vi "Teleop.vi"(10 "Match Info":T2={"Autonomous Elapsed Seconds"=0.0, "TeleOp Elapsed Seconds"=59.421, "Disabled Elapsed Seconds"=50.178, "Visited Autonomous"=FALSE, "Visited TeleOp"=TRUE, "Visited Disabled"=TRUE, "Autonomous Settings"={"Autonomous Style"=enum."Independent", "VI Refnum"=refnum}}, 11 "Call Context":T3=enum."Stop") -> ()   [LabVIEW 2014]
doc: "This VI is called for each TeleOp packet received from the DS where the robot is not disabled. It is often used to read from the joysticks and update I/O or to update setpoints for timed control loops. It should complete and return within 20 milliseconds or it may miss DS packets."
uses:
  <vilib>/Rock Robotics/WPI/DriverStation/WPI_DriverStationDerivedRobotMode.ctl
  <vilib>/Rock Robotics/WPI/DriverStation/WPI_DriverStationMatch Info.ctl
  <vilib>/Rock Robotics/WPI/RobotDrive/WPI_RobotDriveGetSetRefNum.vi
  <vilib>/Rock Robotics/WPI/Joystick/WPI_JoystickGetSetRefNum.vi
  <vilib>/Rock Robotics/Network Tables/SD Write Numeric Array.vi
  <vilib>/Rock Robotics/Network Tables/SD Write Boolean Array.vi
  Robot Global Data.vi
  <vilib>/Rock Robotics/WPI/RobotDrive/WPI_RobotDriveMecanumDrive_Cartesian.vi
panel:
  out "North":dbl
  out "current (A)":dbl(graph)
  in  "Clear Sticky Faults":bool
  in  "PID gains":T1={"proportional gain (Kc)"=0.021, "integral time (Ti, min)"=0.0, "derivative time (Td, min)"=0.0} {"derivative time (Td, min)" format="%.3f"; "integral time (Ti, min)" format="%.3f"; "proportional gain (Kc)" format="%.3f"}
  # "EDITED: 3/8/15"
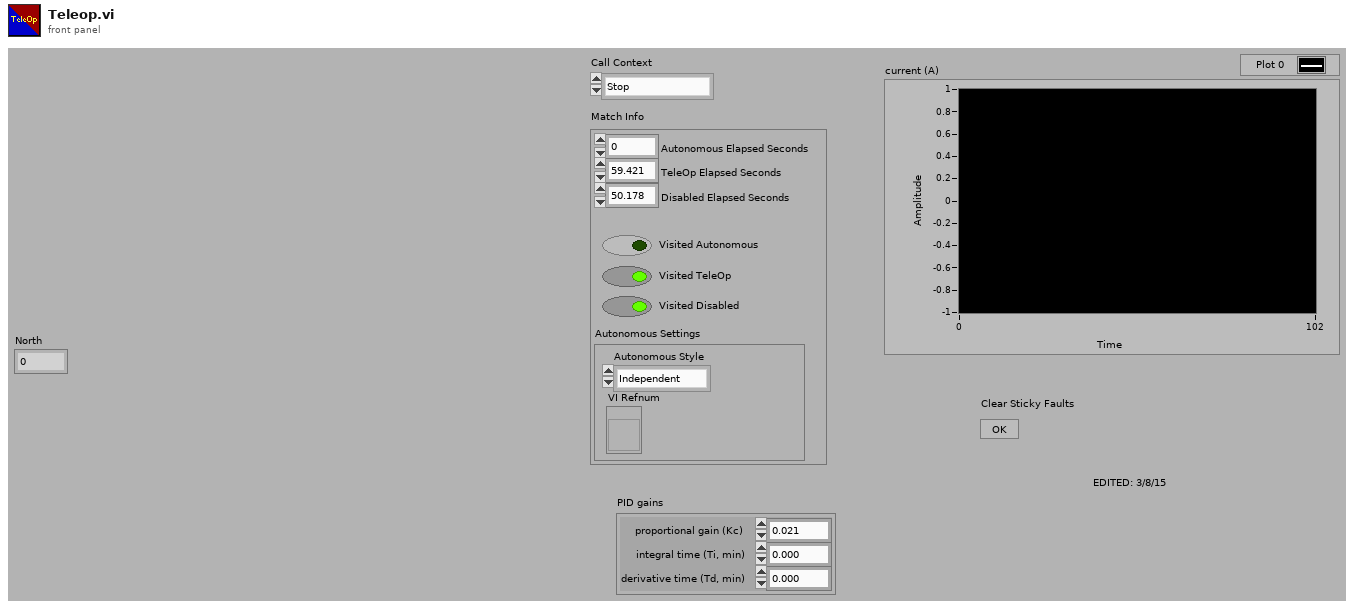
[diagram p1: front panel]
types:
  T1 = cluster{"proportional gain (Kc)":dbl, "integral time (Ti, min)":dbl, "derivative time (Td, min)":dbl}
  T2 = typedef "WPI_DriverStationMatch Info.ctl" = cluster{"Autonomous Elapsed Seconds":dbl, "TeleOp Elapsed Seconds":dbl, "Disabled Elapsed Seconds":dbl, "Visited Autonomous":bool, "Visited TeleOp":bool, "Visited Disabled":bool, "Autonomous Settings":cluster{"Autonomous Style":enum16{"Iterative", "Independent"}, "VI Refnum":refnum<vi>}}
  T3 = typedef "WPI_DriverStationDerivedRobotMode.ctl" = enum16{"Init", "Execute", "Stop"}
  T4 = typedef "WPI_JoystickDevRef.ctl" = cluster{"Device":T5}
  T5 = typedef "WPI_JoystickDeviceEnum.ctl" = enum16{"USB 0", "USB 1", "USB 2", "USB 3", "USB 4", "USB 5"}
  T6 = typedef "WPI_RobotDriveDevRef.ctl" = cluster{"DevStatus":errorcluster, "Motors[]":T7[], "Square Inputs":bool, "Max Output":dbl}
  T7 = typedef "WPI_MotorControlDeviceRef.ctl" = cluster{"DeviceStatus":errorcluster, "Type":T8, "PWM":cluster{"Controller":T9, "PWM Channel":T10, "DeadBand":T11}, "CAN":cluster{"Device Number":u8, "Control Mode":T12, "Semaphore":T13, "Max Vout":dbl, "TalonSRX Control Mode":T14}, "Invert":bool, "TransformRef":T15, "InvTransformRef":T15}
  T8 = typedef "WPI_MotorControlType.ctl" = enum16{"PWM", "CAN", "CANTalonSRX"}
  T9 = typedef "FPGA_TypedefDigitalModule.ctl" = enum16{"Controller 1"}
  T10 = typedef "FPGA_DIOPWMChannel.ctl" = enum8{"PWM 0", "PWM 1", "PWM 2", "PWM 3", "PWM 4", "PWM 5", "PWM 6", "PWM 7", "PWM 8", "PWM 9", "PWM MXP 0", "PWM MXP 1", "PWM MXP 2", "PWM MXP 3", "PWM MXP 4", "PWM MXP 5", "PWM MXP 6", "PWM MXP 7", "PWM MXP 8", "PWM MXP 9", "Invalid"}
  T11 = typedef "WPI_PWMDeadband.ctl" = cluster{"Name":string, "maxPositivePwm":i32, "minPositivePwm":i32, "centerPwm":i32, "maxNegativePwm":i32, "minNegativePwm":i32, "angularRange":u16}
  T12 = typedef "WPI_CANJaguar_ControlMode.ctl" = enum8{"Percent VBus", "Current", "Speed", "Position", "Voltage"}
  T13 = typedef "Semaphore RefNum" = refnum<k1>
  T14 = typedef "WPI_CANTalonSRX_APIControlMode.ctl" = enum8{"Percent VBus", "Speed", "Position", "Slave", "Unchanged / Invalid"}
  T15 = typedef "WPI_PWMTransform_ConPane.ctl" = refnum<vi>
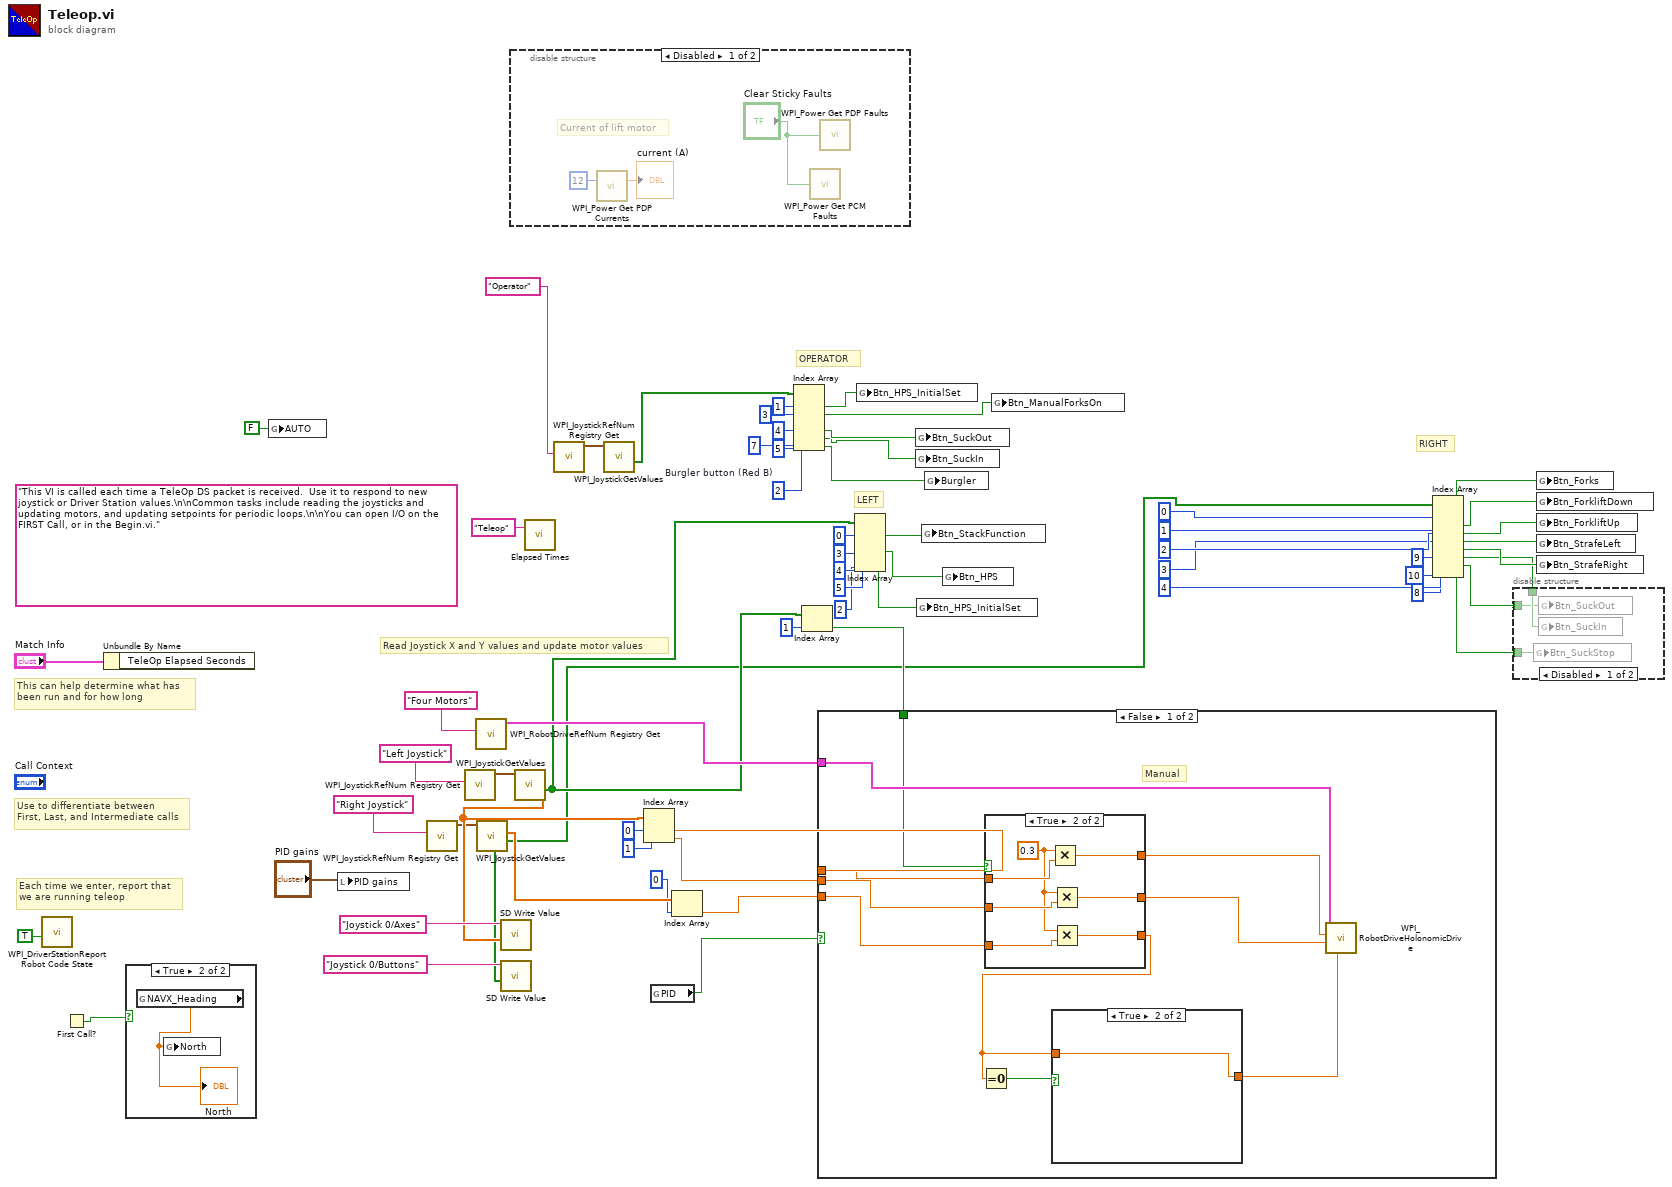
[diagram p0: block diagram]
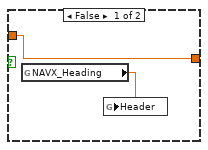
[diagram p5: hidden frame]
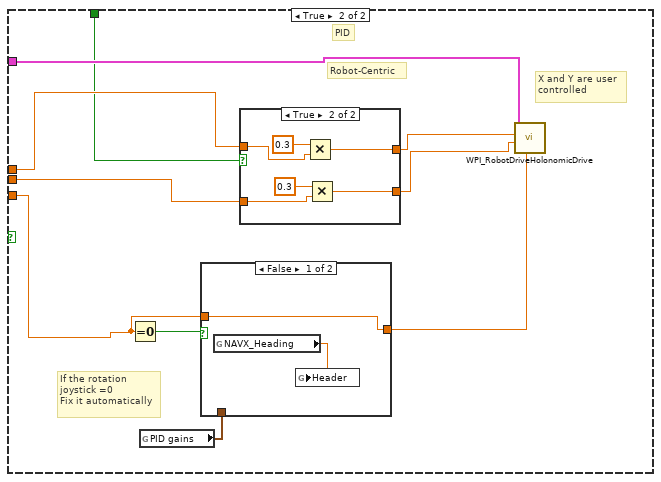
[diagram p7: hidden frame]
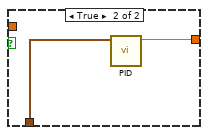
[diagram p8: hidden frame]
diagram:
  w2 = 2  # Burgler button (Red B)
  (unwired) "This VI is called each time a TeleOp DS packet is received.  Use it to respond to new joystick or Driver Station values.\n\nCommon tasks include reading the joysticks and updating motors, and updating setpoints for periodic loops.\n\nYou can open I/O on the FIRST Call, or in the Begin.vi."
  # "LEFT"
  # "OPERATOR"
  # "RIGHT"
  # "Each time we enter, report that\nwe are running teleop"
  # "Use to differentiate between\nFirst, Last, and Intermediate calls"
  # "This can help determine what has\nbeen run and for how long"
  # "Read Joystick X and Y values and update motor values"
  n1 = call <vilib>:"WPI_DriverStationReport Robot Code State.vi"("TeleOp"=TRUE ("Autonomous")) -> ()  [unwired: 10 in, 1 out]
  n2 = First Call?() -> (First Call?: T/F=w7:bool)
  n3 = Unbundle By Name("Match Info") -> ()  [unwired: 1 out]
  n4 = case shown="True" w7 {
    frame False {
    }
    frame True {
      n5 = global read "Robot Global Data.vi" "NAVX_Heading"() -> (w66:dbl)
      "North" <- w66
      n6 = global write "Robot Global Data.vi" "North"(w66) -> ()
    }
  }
  n7 = global write "Robot Global Data.vi" "AUTO"(FALSE ("AUTO")) -> ()
  n8 = local write "PID gains"("PID gains") -> ()
  n9 = call <vilib>:"WPI_JoystickRefNum Registry Get.vi"("refnum name"="Right Joystick") -> ("JoystickDevRef"=w52:T4)  [unwired: 1 in, 9 out]
  n10 = call <vilib>:"WPI_JoystickRefNum Registry Get.vi"("refnum name"="Left Joystick") -> ("JoystickDevRef"=w62:T4)  [unwired: 1 in, 9 out]
  n11 = call <vilib>:"WPI_RobotDriveRefNum Registry Get.vi"("refnum name"="Four Motors") -> ("RobotDriveDevRef"=w53:T6)  [unwired: 1 in, 9 out]
  n12 = call <vilib>:"WPI_JoystickGetValues.vi"("JoystickDevRef"=w52) -> ("Buttons"=w25:bool[], "Axes"=w50:dbl[])  [unwired: 6 in, 3 out]
  n13 = call-poly <vilib>:"SD Write Value.vi"("Boolean Array"=w25, "Name"="Joystick 0/Buttons") -> ()  [unwired: 8 in, 2 out]
  n14 = disable-structure shown="Disabled" {
    frame Disabled {
      # "Current of lift motor"
      n15 = call <vilib>:"WPI_Power Get PDP Currents.vi"("PDP Channel"=12) -> ("current (A)"=→"current (A)":dbl)  [unwired: 12 in, 2 out]
      n16 = call <vilib>:"WPI_Power Get PCM Faults.vi"("Clear Sticky Faults"="Clear Sticky Faults") -> ()  [unwired: 11 in, 4 out]
      n17 = call <vilib>:"WPI_Power Get PDP Faults.vi"("Clear Sticky Faults"="Clear Sticky Faults") -> ()  [unwired: 10 in, 5 out]
    }
    frame Enabled {
    }
  }
  n18 = call <vilib>:"WPI_JoystickGetValues.vi"("JoystickDevRef"=w62) -> ("Buttons"=w45:bool[], "Axes"=w58:dbl[])  [unwired: 6 in, 3 out]
  n19 = call-poly <vilib>:"SD Write Value.vi"("Numeric Array"=w58, "Name"="Joystick 0/Axes") -> ()  [unwired: 8 in, 2 out]
  n20 = call "Elapsed Times.vi"("Call Name"="Teleop") -> ()  [unwired: 2 in, 1 out]
  n21 = call <vilib>:"WPI_JoystickRefNum Registry Get.vi"("refnum name"="Operator") -> ("JoystickDevRef"=w28:T4)  [unwired: 1 in, 9 out]
  n22 = call <vilib>:"WPI_JoystickGetValues.vi"("JoystickDevRef"=w28) -> ("Buttons"=w26:bool[])  [unwired: 6 in, 4 out]
  n23 = Index Array(array=w58, index #1=0 ("index"), index #2=1 ("index")) -> (element #1=w55:dbl, element #2=w54:dbl)
  n24 = global read "Robot Global Data.vi" "PID"() -> (w6:bool)
  n25 = Index Array(array=w50, index=0) -> (element=w48:dbl)
  n26 = Index Array(array=w26, index #1=1 ("index"), index #2=3 ("index"), index #3=7 ("index"), index #4=4 ("index"), index #5=5 ("index"), index #6=w2) -> (element #1=w22:bool, element #2=w21:bool, element #4=w11:bool, element #5=w10:bool, element #6=w1:bool)  [unwired: 1 out]
  n27 = Index Array(array=w45, index=1) -> (element=w46:bool)
  n28 = case shown="False" w6 {
    tunnel: w55 -> [w79 w102]
    tunnel: w54 -> [w78 w101]
    tunnel: w48 -> [w74 w94]
    tunnel: w53 -> [w77 w100]
    tunnel: w46 -> [w73 w99]
    frame False {
      # "Manual"
      n29 = case shown="True" w73 {
        tunnel: [w85 w92] -> w76
        tunnel: [w84 w91] -> w75
        tunnel: w79 -> [w85 w90]
        tunnel: w78 -> [w84 w89]
        tunnel: w74 -> [w83 w88]
        tunnel: [w83 w87] -> w71
        frame False {
        }
        frame True {
          w86 = 0.3 ("x")
          n30 = Multiply(x=w86, y=w90) -> (x*y=w92:dbl)
          n31 = Multiply(x=w86, y=w89) -> (x*y=w91:dbl)
          n32 = Multiply(x=w86, y=w88) -> (x*y=w87:dbl)
        }
      }
      n33 = Equal To 0?(x=w71) -> (x = 0?=w72:bool)
      n34 = case shown="True" w72 {
        tunnel: [w80 w82] -> w70
        tunnel: w71 -> [w80 w82]
        frame False {
          n35 = global read "Robot Global Data.vi" "NAVX_Heading"() -> (w81:dbl)
          n36 = global write "Robot Global Data.vi" "Header"(w81) -> ()
        }
        frame True {
        }
      }
      n37 = call-poly <vilib>:"WPI_RobotDriveHolonomicDrive.vi"("Rotation"=w70, "Y"=w75, "X"=w76, "RobotDriveDevRef"=w77) -> ()  [unwired: 5 in, 3 out]
    }
    frame True {
      # "If the rotation\njoystick =0\nFix it automatically"
      # "X and Y are user \ncontrolled"
      # "Robot-Centric"
      # "PID"
      n38 = Equal To 0?(x=w94) -> (x = 0?=w95:bool)
      n39 = global read "Robot Global Data.vi" "PID gains"() -> (w93:T1)
      n40 = case shown="False" w95 {
        tunnel: [w104 w106] -> w98
        tunnel: w94 -> [w104 _]
        tunnel: w93 -> [_ w105]
        frame False {
          n41 = global read "Robot Global Data.vi" "NAVX_Heading"() -> (w103:dbl)
          n42 = global write "Robot Global Data.vi" "Header"(w103) -> ()
        }
        frame True {
          n43 = call "PID.vi"("PID gains"=w105) -> ("output"=w106:dbl)  [unwired: 10 in]
        }
      }
      n44 = case shown="True" w99 {
        tunnel: [w108 w112] -> w97
        tunnel: [w107 w111] -> w96
        tunnel: w102 -> [w108 w110]
        tunnel: w101 -> [w107 w109]
        frame False {
        }
        frame True {
          n45 = Multiply(x=0.3, y=w110) -> (x*y=w112:dbl)
          n46 = Multiply(x=0.3, y=w109) -> (x*y=w111:dbl)
        }
      }
      n47 = call-poly <vilib>:"WPI_RobotDriveHolonomicDrive.vi"("Rotation"=w98, "Y"=w96, "X"=w97, "RobotDriveDevRef"=w100) -> ()  [unwired: 5 in, 3 out]
    }
  }
  n48 = Index Array(array=w45, index #1=0 ("index"), index #2=3 ("index"), index #3=4 ("index"), index #4=5 ("index"), index #5=2 ("index")) -> (element #1=w43:bool, element #3=w30:bool, element #5=w14:bool)  [unwired: 2 out]
  n49 = global write "Robot Global Data.vi" "Btn_HPS_InitialSet"(w22) -> ()
  n50 = global write "Robot Global Data.vi" "Btn_SuckOut"(w11) -> ()
  n51 = global write "Robot Global Data.vi" "Btn_SuckIn"(w10) -> ()
  n52 = global write "Robot Global Data.vi" "Btn_HPS_InitialSet"(w14) -> ()
  n53 = global write "Robot Global Data.vi" "Btn_StackFunction"(w43) -> ()
  n54 = global write "Robot Global Data.vi" "Burgler"(w1) -> ()
  n55 = global write "Robot Global Data.vi" "Btn_HPS"(w30) -> ()
  n56 = global write "Robot Global Data.vi" "Btn_ManualForksOn"(w21) -> ()
  n57 = Index Array(array=w25, index #1=0 ("index"), index #2=1 ("index"), index #3=2 ("index"), index #4=3 ("index"), index #5=4 ("index"), index #6=9 ("index"), index #7=10 ("index"), index #8=8 ("index")) -> (element #1=w42:bool, element #2=w38:bool, element #3=w37:bool, element #4=w36:bool, element #5=w35:bool, element #6=w18:bool, element #7=w17:bool, element #8=w3:bool)
  n58 = disable-structure shown="Disabled" {
    disable-tunnel: w18 -> [w117 _]
    disable-tunnel: w17 -> [w116 _]
    disable-tunnel: w3 -> [w115 _]
    frame Disabled {
      n59 = global write "Robot Global Data.vi" "Btn_SuckStop"(w115) -> ()
      n60 = global write "Robot Global Data.vi" "Btn_SuckOut"(w116) -> ()
      n61 = global write "Robot Global Data.vi" "Btn_SuckIn"(w117) -> ()
    }
    frame Enabled {
    }
  }
  n62 = global write "Robot Global Data.vi" "Btn_Forks"(w42) -> ()
  n63 = global write "Robot Global Data.vi" "Btn_ForkliftDown"(w38) -> ()
  n64 = global write "Robot Global Data.vi" "Btn_ForkliftUp"(w37) -> ()
  n65 = global write "Robot Global Data.vi" "Btn_StrafeLeft"(w36) -> ()
  n66 = global write "Robot Global Data.vi" "Btn_StrafeRight"(w35) -> ()
